vi "GetDescription.vi"(8 "error in (no error)":errorcluster caption="错误输入（无错误）", 11 "Mocha 输入":refnum<class "Mocha.lvclass">) -> (0 "error out":errorcluster caption="错误输出", 2 "Description":string, 3 "Mocha 输出":refnum<class "Mocha.lvclass">)   [LabVIEW 2016, in "Mocha.lvclass"]
uses:
  Mocha.lvclass
  Mocha.lvclass/Mocha.ctl
  CondimentDecorator.lvclass
  Beverage.lvclass
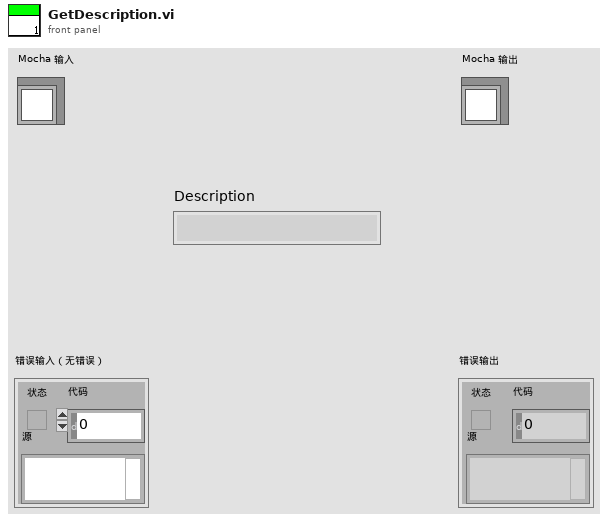
[diagram p1: front panel]
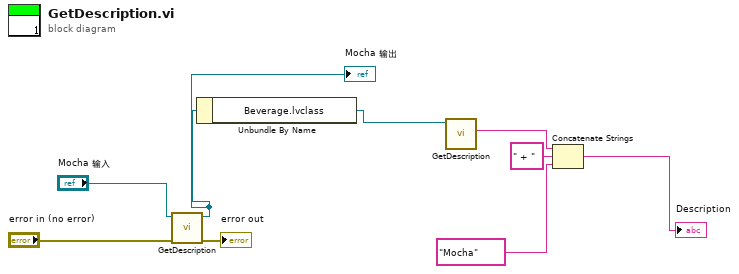
[diagram p0: block diagram]
diagram:
  n1 = call-parent "GetDescription.vi"("error in (no error)"="error in (no error)", "CondimentDecorator 输入"="Mocha 输入") -> ("error out"=→"error out":errorcluster, "CondimentDecorator 输出"=w6:refnum<class "Mocha.lvclass">)  [unwired: 7 in, 1 out]
  "Mocha 输出" <- w6
  n2 = Unbundle By Name(w6) -> ("Beverage.lvclass"=w5:refnum<class "Beverage.lvclass">)
  n3 = call-dynamic "GetDescription.vi"("Beverage 输入"=w5) -> ("Description"=w4:string)  [unwired: 8 in, 2 out]
  n4 = Concatenate Strings(w4, " + " ("字符串"), "Mocha" ("Description")) -> (→"Description":string)
